vi "SwerveDrivePoseEst2_AddVisionMeasurement.vi"(9 "TImeStamp_Seconds":dbl=0.02, 10 "visionRobotPose":T9={"TRANSLATION"={"X"=0.0, "Y"=0.0}, "ROTATION"={"VALUE"=0.0, "COS"=1.0, "SIN"=0.0}} {"ROTATION"."SIN" format="%13.4f"; "ROTATION"."COS" format="%13.4f"; "ROTATION"."VALUE" format="%13.4f"; "TRANSLATION"."Y" format="%14.3f"; "TRANSLATION"."X" format="%14.3f"}, 11 "in SwerveDrivePoseEst2":T1={"M_Vision_K"=[], "m_nominal_dT"=0.0, "m_PrevTime_Sec"=0.0, "Pose_Buffer"={"TimeStamps"=[], "DataArray"=[], "Min_TimeStamp"=0.0, "Max_TimeStamp"=0.0, "ItemCount"=0, "MaxBufferTime"=0.0}, "Swerve_Drive_Kinematics"={"NumModules"=0, "InverseKinematics"=[], "ForwardKinematics"=[], "Modules"=[], "PrevCoR"={"X"=0.0, "Y"=0.0}, "SavedModuleStates"=[]}, "Swerve_Drive_Odom"={"POSE"={"TRANSLATION"={"X"=0.0, "Y"=0.0}, "ROTATION"={"VALUE"=0.0, "COS"=1.0, "SIN"=0.0}}, "GyroOffset"={"VALUE"=0.0, "COS"=1.0, "SIN"=0.0}, "PreviousAngle"={"VALUE"=0.0, "COS"=1.0, "SIN"=0.0}, "PrevModulePositions"=[], "NumModules"=0}, "M_Q"=[[0.0], [0.0], [0.0]], "NumModules"=-1} {"Swerve_Drive_Odom"."PrevModulePositions"."Angle"."SIN" format="%13.4f"; "Swerve_Drive_Odom"."PrevModulePositions"."Angle"."COS" format="%13.4f"; "Swerve_Drive_Odom"."PrevModulePositions"."Angle"."VALUE" format="%13.4f"; "Swerve_Drive_Odom"."PreviousAngle"."SIN" format="%13.4f"; "Swerve_Drive_Odom"."PreviousAngle"."COS" format="%13.4f"; "Swerve_Drive_Odom"."PreviousAngle"."VALUE" format="%13.4f"; "Swerve_Drive_Odom"."GyroOffset"."SIN" format="%13.4f"; "Swerve_Drive_Odom"."GyroOffset"."COS" format="%13.4f"; "Swerve_Drive_Odom"."GyroOffset"."VALUE" format="%13.4f"; "Swerve_Drive_Odom"."POSE"."ROTATION"."SIN" format="%13.4f"; "Swerve_Drive_Odom"."POSE"."ROTATION"."COS" format="%13.4f"; "Swerve_Drive_Odom"."POSE"."ROTATION"."VALUE" format="%13.4f"; "Swerve_Drive_Odom"."POSE"."TRANSLATION"."Y" format="%14.3f"; "Swerve_Drive_Odom"."POSE"."TRANSLATION"."X" format="%14.3f"; "Swerve_Drive_Kinematics"."SavedModuleStates"."Angle"."SIN" format="%13.4f"; "Swerve_Drive_Kinematics"."SavedModuleStates"."Angle"."COS" format="%13.4f"; "Swerve_Drive_Kinematics"."SavedModuleStates"."Angle"."VALUE" format="%13.4f"; "Swerve_Drive_Kinematics"."PrevCoR"."Y" format="%14.3f"; "Swerve_Drive_Kinematics"."PrevCoR"."X" format="%14.3f"; "Swerve_Drive_Kinematics"."Modules"."Y" format="%14.3f"; "Swerve_Drive_Kinematics"."Modules"."X" format="%14.3f"}) -> (0 "Error":bool, 3 "Out SwerveDrivePoseEst2":T1={"M_Vision_K"=[], "m_nominal_dT"=0.0, "m_PrevTime_Sec"=0.0, "Pose_Buffer"={"TimeStamps"=[], "DataArray"=[], "Min_TimeStamp"=0.0, "Max_TimeStamp"=0.0, "ItemCount"=0, "MaxBufferTime"=0.0}, "Swerve_Drive_Kinematics"={"NumModules"=0, "InverseKinematics"=[], "ForwardKinematics"=[], "Modules"=[], "PrevCoR"={"X"=0.0, "Y"=0.0}, "SavedModuleStates"=[]}, "Swerve_Drive_Odom"={"POSE"={"TRANSLATION"={"X"=0.0, "Y"=0.0}, "ROTATION"={"VALUE"=0.0, "COS"=1.0, "SIN"=0.0}}, "GyroOffset"={"VALUE"=0.0, "COS"=1.0, "SIN"=0.0}, "PreviousAngle"={"VALUE"=0.0, "COS"=1.0, "SIN"=0.0}, "PrevModulePositions"=[], "NumModules"=0}, "M_Q"=[[0.0], [0.0], [0.0]], "NumModules"=-1} {"Swerve_Drive_Odom"."PrevModulePositions"."Angle"."SIN" format="%13.4f"; "Swerve_Drive_Odom"."PrevModulePositions"."Angle"."COS" format="%13.4f"; "Swerve_Drive_Odom"."PrevModulePositions"."Angle"."VALUE" format="%13.4f"; "Swerve_Drive_Odom"."PreviousAngle"."SIN" format="%13.4f"; "Swerve_Drive_Odom"."PreviousAngle"."COS" format="%13.4f"; "Swerve_Drive_Odom"."PreviousAngle"."VALUE" format="%13.4f"; "Swerve_Drive_Odom"."GyroOffset"."SIN" format="%13.4f"; "Swerve_Drive_Odom"."GyroOffset"."COS" format="%13.4f"; "Swerve_Drive_Odom"."GyroOffset"."VALUE" format="%13.4f"; "Swerve_Drive_Odom"."POSE"."ROTATION"."SIN" format="%13.4f"; "Swerve_Drive_Odom"."POSE"."ROTATION"."COS" format="%13.4f"; "Swerve_Drive_Odom"."POSE"."ROTATION"."VALUE" format="%13.4f"; "Swerve_Drive_Odom"."POSE"."TRANSLATION"."Y" format="%14.3f"; "Swerve_Drive_Odom"."POSE"."TRANSLATION"."X" format="%14.3f"; "Swerve_Drive_Kinematics"."SavedModuleStates"."Angle"."SIN" format="%13.4f"; "Swerve_Drive_Kinematics"."SavedModuleStates"."Angle"."COS" format="%13.4f"; "Swerve_Drive_Kinematics"."SavedModuleStates"."Angle"."VALUE" format="%13.4f"; "Swerve_Drive_Kinematics"."PrevCoR"."Y" format="%14.3f"; "Swerve_Drive_Kinematics"."PrevCoR"."X" format="%14.3f"; "Swerve_Drive_Kinematics"."Modules"."Y" format="%14.3f"; "Swerve_Drive_Kinematics"."Modules"."X" format="%14.3f"})   [LabVIEW 2019, in "Trajectory_Library.lvlib"]
doc: "Add a vision measurement to the Unscented Kalman Filter. This will correct the odometry pose estimate while still accounting for measurement noise.\n \nThis method can be called as infrequently as you want, as long as you are calling SwerveDrivePoseEstimator_update every loop.\n\nTo promote stability of the pose estimate and make it robust to bad vision data, we recommend only adding vision measurements that are already within one meter or so of the current pose estimate.\n\n Inputs:\n - InSwerveDrivePoseEstimate -- Data cluster for this system\n - visionRobotPoseMeters -- The pose of the robot as measured by the vision camera.\n - timestampSeconds -- The timestamp of the vision measurement in seconds. Note that if you don't use your own time source by calling SwerveDrivePoseEstimator_updateWithTime then you must use a timestamp with an epoch since FPGA startup (i.e. the epoch of this timestamp is the same epoch as Util_GetFPGATime.) This means that you should use Util_GetFPGATime as your time source in this case.\n\nOutputs:\n - OutSwerveDrivePoseEstimate2 -- Data cluster for this system\n - Error -- Returns TRUE if an error occured."
uses:
  Trajectory_Library.lvlib
  TypeDef/SWERVE_DRIVE_POSE_EST2.ctl
  <vilib>/Analysis/Matrix/Datatypes/RealMatrix.ctl
  TypeDef/TIME_INTERPOLATABLE_VARIANT.ctl
  TypeDef/SWERVE_DRIVE_KINEMATICS.ctl
  TypeDef/TRANSLATION2D.ctl
  TypeDef/SWERVE_DRIVE_MODULE_STATE.ctl
  TypeDef/ROTATION2D.ctl
  TypeDef/SWERVE_DRIVE_ODOMETRY.ctl
  TypeDef/POSE2D.ctl
  TypeDef/SWERVE_DRIVE_MODULE_POSITION.ctl
  <vilib>/Analysis/baseanly.llb/Real A x B.vi
  MatBuilder_Create.vi
  Pose2d_getRotation.vi
  Rotation2d_Minus.vi
  TimeInterpVariant_CleanUp.vi
  Rotation2d_UnaryMinus.vi
  Rotation2d_RotateBy.vi
  Rotation2d_CreateAngle.vi
  Rotation2d_CreateXY.vi
  Util_CalcDist.vi
  SwerveDrivePoseEst2_InterpRecord_Interp.vi
  <vilib>/gmath/interp.llb/Search Ordered Table.vi
  <vilib>/Analysis/NI_AALBase.lvlib
  <vilib>/Analysis/Matrix/NI_Matrix.lvlib
panel:
  # "<3, 1>"
  # "<3, 3>"
  # "<3, 1>"
  # "<3, 3>"
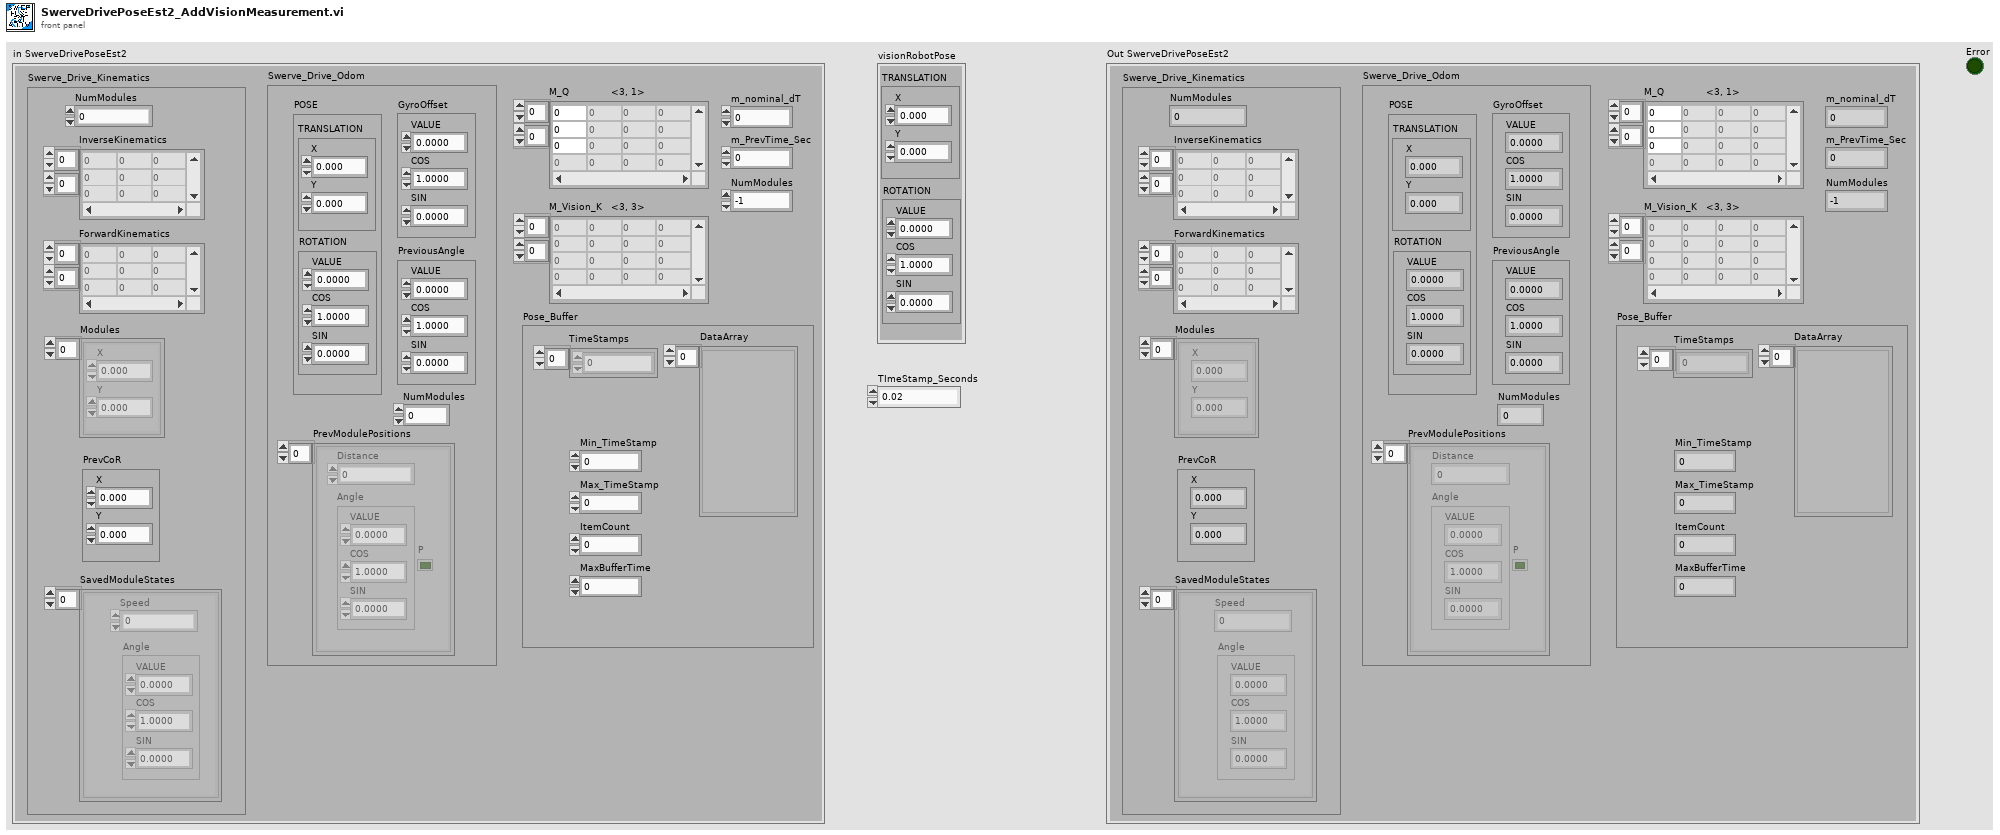
[diagram p1: front panel]
types:
  T1 = typedef "Trajectory_Library.lvlib/SWERVE_DRIVE_POSE_EST2.ctl" = cluster{"M_Vision_K":T2, "m_nominal_dT":dbl, "m_PrevTime_Sec":dbl, "Pose_Buffer":T3, "Swerve_Drive_Kinematics":T4, "Swerve_Drive_Odom":T8, "M_Q":T2, "NumModules":i32}
  T2 = typedef "NI_Matrix.lvlib/RealMatrix.ctl" = dbl[][]
  T3 = typedef "Trajectory_Library.lvlib/TIME_INTERPOLATABLE_VARIANT.ctl" = cluster{"TimeStamps":dbl[], "DataArray":variant[], "Min_TimeStamp":dbl, "Max_TimeStamp":dbl, "ItemCount":i32, "MaxBufferTime":dbl}
  T4 = typedef "Trajectory_Library.lvlib/SWERVE_DRIVE_KINEMATICS.ctl" = cluster{"NumModules":i32, "InverseKinematics":T2, "ForwardKinematics":T2, "Modules":T5[], "PrevCoR":T5, "SavedModuleStates":T6[]}
  T5 = typedef "Trajectory_Library.lvlib/TRANSLATION2D.ctl" = cluster{"X":dbl, "Y":dbl}
  T6 = typedef "Trajectory_Library.lvlib/SWERVE_DRIVE_MODULE_STATE.ctl" = cluster{"Speed":dbl, "Angle":T7}
  T7 = typedef "Trajectory_Library.lvlib/ROTATION2D.ctl" = cluster{"VALUE":dbl, "COS":dbl, "SIN":dbl}
  T8 = typedef "Trajectory_Library.lvlib/SWERVE_DRIVE_ODOMETRY.ctl" = cluster{"POSE":T9, "GyroOffset":T7, "PreviousAngle":T7, "PrevModulePositions":T10[], "NumModules":i32}
  T9 = typedef "Trajectory_Library.lvlib/POSE2D.ctl" = cluster{"TRANSLATION":T5, "ROTATION":T7}
  T10 = typedef "Trajectory_Library.lvlib/SWERVE_DRIVE_MODULE_POSITION.ctl" = cluster{"Distance":dbl, "Angle":T7, "P":bool}
  T11 = typedef "Trajectory_Library.lvlib/SWERVE_DRIVE_POSE_EST2_INTERP_RECORD.ctl" = cluster{"PoseMeters":T9, "GyroAngle":T7, "ModulePositions":T10[]}
  T12 = typedef "Trajectory_Library.lvlib/TWIST2D.ctl" = cluster{"dX":dbl, "dY":dbl, "dTHETA":dbl}
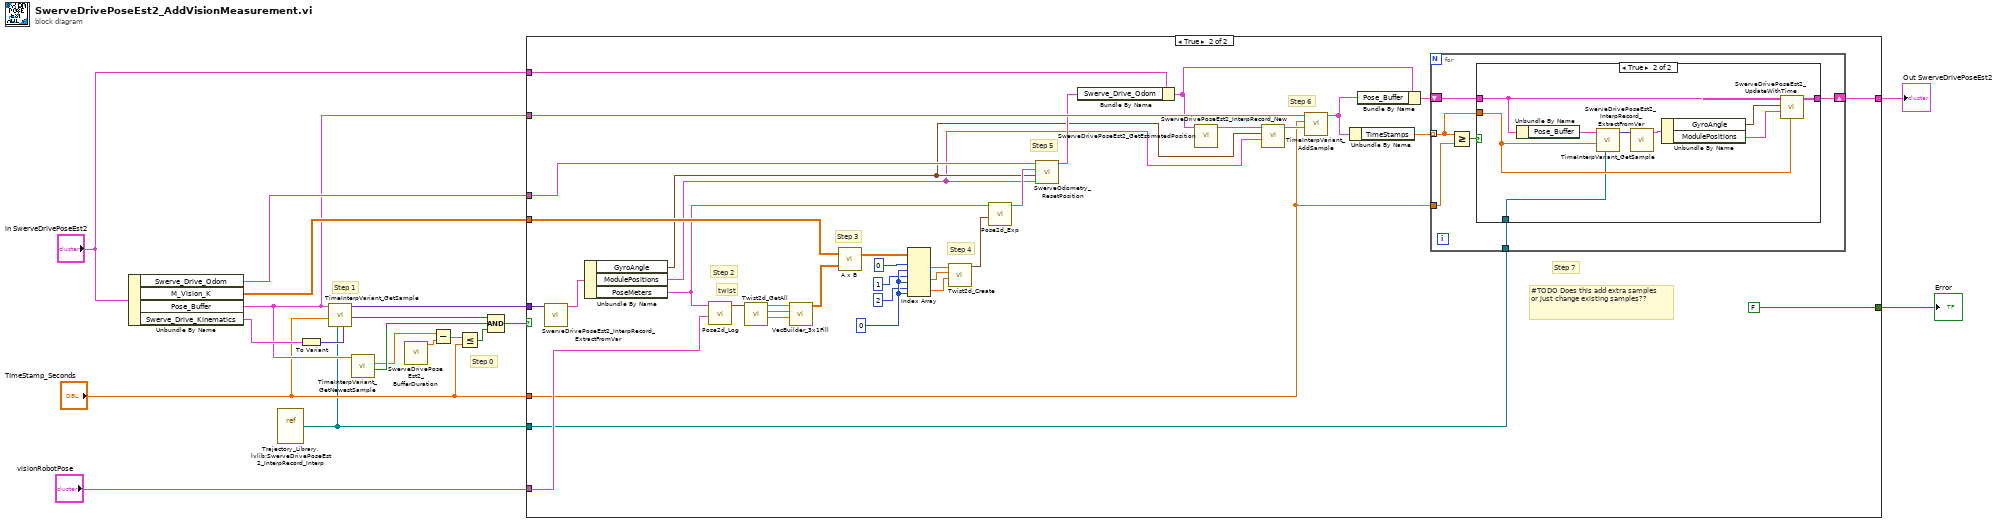
[diagram p0: block diagram]
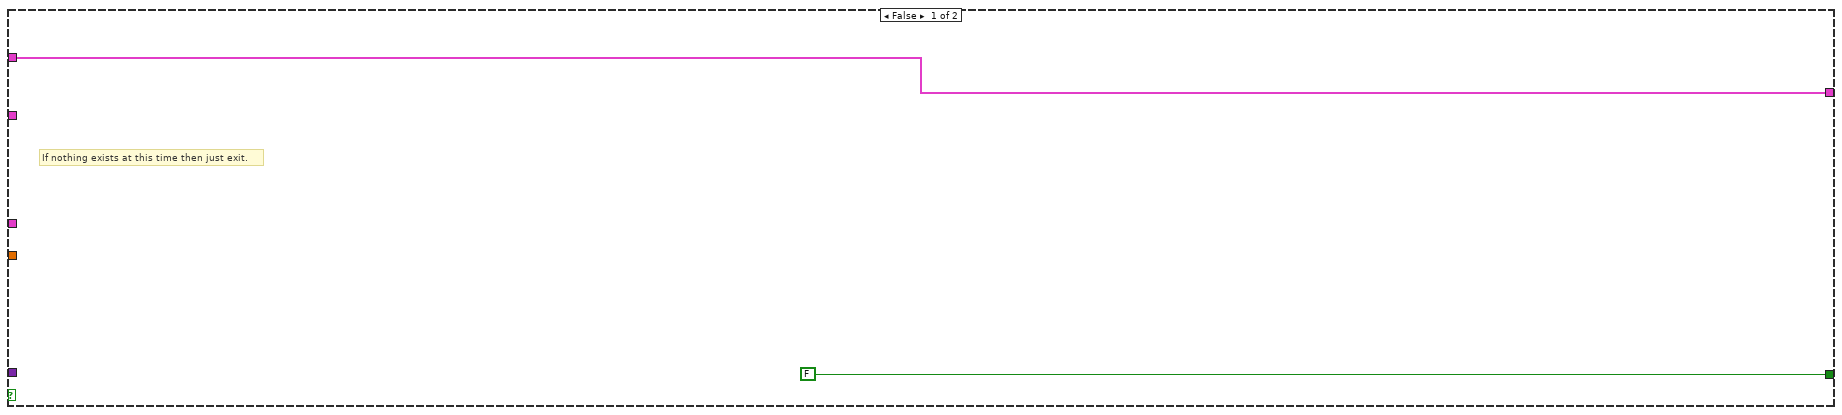
[diagram p2: hidden frame]
diagram:
  # "Step 0"
  # "Step 1"
  n1 = Unbundle By Name("in SwerveDrivePoseEst2") -> ("Swerve_Drive_Odom"=w11:T8, "M_Vision_K"=w12:T2, "Pose_Buffer"=w10:T3, "Swerve_Drive_Kinematics"=w14:T4)
  n2 = vi-ref "Trajectory_Library.lvlib:SwerveDrivePoseEst2_InterpRecord_Interp.vi"() -> (w1:refnum<vi>)
  n3 = To Variant(anything=w14) -> (Variant=w15:variant)
  n4 = call "TimeInterpVariant_GetSample.vi"("Extra"=w15, "Interpolate\nReference"=w1, "TimeStamp"="TImeStamp_Seconds", "TimeInterpVariant"=w10) -> ("IsPresent"=w9:bool, "OutputVariant"=w13:variant)  [unwired: 6 in]
  n5 = call "TimeInterpVariant_GetNewestSample.vi"("TimeInterpVariant"=w10) -> ("IsPresent"=w8:bool, "TimeStamp"=w7:dbl)  [unwired: 8 in, 1 out]
  n6 = call "SwerveDrivePoseEst2_BufferDuration.vi"() -> ("Buffer Duration (Sec)"=w3:dbl)  [unwired: 11 in]
  n7 = Subtract(x=w7, y=w3) -> (x-y=w6:dbl)
  n8 = Less Or Equal?(x=w6, y="TImeStamp_Seconds") -> (x <= y?=w5:bool)
  n9 = Compound Arithmetic op=AND(w9, w8, w5) -> (w4:bool)
  n10 = case shown="True" w4 {
    tunnel: [w21 w26] -> w19
    tunnel: "visionRobotPose" -> [_ w55]
    tunnel: [FALSE FALSE] -> w17
    tunnel: "in SwerveDrivePoseEst2" -> [w21 w34]
    tunnel: w13 -> [_ w57]
    tunnel: w12 -> [_ w54]
    tunnel: w11 -> [_ w40]
    tunnel: w10 -> [_ w36]
    tunnel: "TImeStamp_Seconds" -> [_ w30]
    tunnel: w1 -> [_ w24]
    frame False {
      # "If nothing exists at this time then just exit."
    }
    frame True {
      w47 = 0 ("index (col)")
      # "#TODO Does this add extra samples\nor just change existing samples??"
      # "Step 7"
      # "Step 6"
      # "Step 5"
      # "Step 4"
      # "Step 3"
      # "twist"
      # "Step 2"
      n11 = call "SwerveDrivePoseEst2_InterpRecord_ExtractFromVar.vi"("OutputVariant"=w57) -> ("out InterpRecord"=w56:T11)  [unwired: 9 in, 1 out]
      n12 = Unbundle By Name(w56) -> ("GyroAngle"=w23:T7, "ModulePositions"=w22:T10[], "PoseMeters"=w39:T9)
      n13 = call "Pose2d_Log.vi"("end POSE"=w55, "in POSE"=w39) -> ("out TWIST"=w53:T12)  [unwired: 9 in]
      n14 = call "Twist2d_GetAll.vi"("TWIST"=w53) -> ("dTHETA"=w50:dbl, "dY"=w51:dbl, "dX"=w52:dbl)  [unwired: 8 in]
      n15 = call "VecBuilder_3x1Fill.vi"("R2"=w50, "R1"=w51, "R0"=w52) -> ("output matrix"=w49:T2)  [unwired: 8 in]
      n16 = call-poly <vilib>:"A x B.vi"("B"=w49, "A"=w54) -> ("A x B"=w48:T2)  [unwired: 1 out]
      n17 = Index Array(array=w48, index (row) #1=0 ("index (row)"), index (col) #1=w47, index (row) #2=1 ("index (row)"), index (col) #2=w47, index (row) #3=2 ("index (row)"), index (col) #3=w47) -> (element #1=w43:dbl, element #2=w42:dbl, element #3=w41:dbl)
      n18 = call "Twist2d_Create.vi"("dTHETA"=w41, "dY"=w42, "dX"=w43) -> ("TWIST"=w38:T12)  [unwired: 8 in]
      n19 = call "Pose2d_Exp.vi"("TWIST"=w38, "POSE"=w39) -> ("UpdatedPose"=w37:T9)  [unwired: 9 in]
      n20 = call "SwerveOdometry_ResetPosition.vi"("Module Positions"=w22, "gyroAngle"=w23, "Pose"=w37, "in SWERVE_DRIVE_ODOMETRY"=w40) -> ("out SWERVE_DRIVE_ODOMETRY"=w33:T8)  [unwired: 6 in, 1 out]
      n21 = Bundle By Name(cluster=w34, "Swerve_Drive_Odom"=w33) -> (w29:T1)
      n22 = call "SwerveDrivePoseEst2_GetEstimatedPosition.vi"("in SwerveDrivePoseEstimate"=w29) -> ("Estimated Pose"=w32:T9)  [unwired: 10 in]
      n23 = call "SwerveDrivePoseEst2_InterpRecord_New.vi"("ModulePositions"=w22, "GyroAngle"=w23, "M_POSE_Meters"=w32) -> ("SWERVE_DRIVE_POSE_EST2_INTERP_RECORD"=w35:T11)  [unwired: 8 in]
      n24 = call "TimeInterpVariant_AddSample.vi"("Variant"=w35, "TimeStamp"=w30, "in TimeInterpVariant"=w36) -> ("out TimeInterpVariant"=w28:T3)  [unwired: 7 in, 1 out]
      n25 = Unbundle By Name(w28) -> ("TimeStamps"=w31:dbl[])
      n26 = Bundle By Name(cluster=w29, "Pose_Buffer"=w28) -> (w27:T1)
      n27 = for {
        tunnel: w31 -> [w62] mode=indexing
        tunnel: w30 -> [w59]
        shift-right: [w60] -> w26
        shift-left: w27 -> [w61]
        tunnel: w24 -> [w58]
        n28 = Greater Or Equal?(x=w62, y=w59) -> (x >= y?=w63:bool)
        n29 = case shown="True" w63 {
          tunnel: w62 -> [_ w67]
          tunnel: w61 -> [w64 w70]
          tunnel: [w64 w73] -> w60
          tunnel: w58 -> [_ w66]
          frame False {
          }
          frame True {
            n30 = Unbundle By Name(w70) -> ("Pose_Buffer"=w69:T3)
            n31 = call "TimeInterpVariant_GetSample.vi"("Extra"=w67, "Interpolate\nReference"=w66, "TimeStamp"=w67, "TimeInterpVariant"=w69) -> ("OutputVariant"=w68:variant)  [unwired: 6 in, 1 out]
            n32 = call "SwerveDrivePoseEst2_InterpRecord_ExtractFromVar.vi"("OutputVariant"=w68) -> ("out InterpRecord"=w72:T11)  [unwired: 9 in, 1 out]
            n33 = Unbundle By Name(w72) -> ("GyroAngle"=w71:T7, "ModulePositions"=w65:T10[])
            n34 = call "SwerveDrivePoseEst2_UpdateWithTime.vi"("CurrentTimeSeconds"=w67, "module Positions"=w65, "GyroAngle"=w71, "in SwerveDrivePoseEst2"=w70) -> ("Out SwerveDrivePoseEst2"=w73:T1)  [unwired: 5 in, 2 out]
          }
        }
      }
    }
  }
  "Out SwerveDrivePoseEst2" <- w19
  "Error" <- w17
